vi "source path to dest txt path.vi"(10 "Source Path":path, 11 "Dest Folder":path) -> (3 "Dest Path":path)   [LabVIEW 2022 SP3]
uses:
  <userlib>/_OpenG.lib/file/file.llb/Convert File Extension (Path)__ogtk.vi
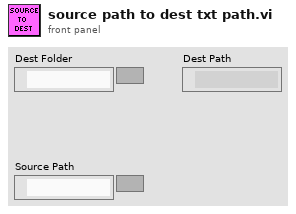
[diagram p1: front panel]
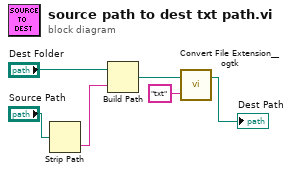
[diagram p0: block diagram]
diagram:
  n1 = Strip Path(path="Source Path") -> (name=w4:string)  [unwired: 1 out]
  n2 = Build Path(base path="Dest Folder", name or relative path=w4) -> (appended path=w2:path)
  n3 = call-poly <userlib>:"Convert File Extension__ogtk.vi"("new ending (none)"="txt", "file name"=w2) -> ("new filename"=→"Dest Path":path)  [unwired: 1 out]
